vi "getPackageFolder.vi"() -> (0 "packageDirectory":path)   [LabVIEW 2023]
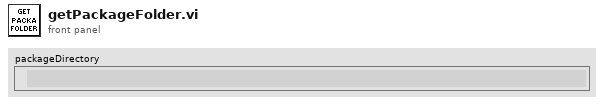
[diagram p1: front panel]
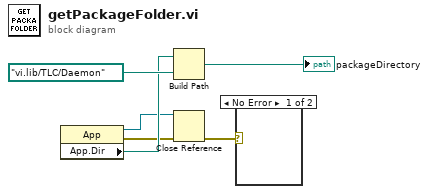
[diagram p0: block diagram]
diagram:
  n1 = property class="App"() -> (reference out=w3:refnum<vi>, error out=w2:errorcluster, "App.Dir"=w4:path)  [unwired: 2 in]
  n2 = Build Path(base path=w4, name or relative path=path "vi.lib/TLC/Daemon") -> (appended path=→"packageDirectory":path)
  n3 = Close Reference(reference=w3, error in (no error)=w2) -> (error out=w1:errorcluster)
  n4 = case shown="No Error" w1 {
    frame No Error {
    }
    frame Error {
    }
  }
